vi "Test - Evaluation and Decoding.vi"() -> ()   [LabVIEW 2014, in "HMM.lvlib"]
uses:
  HMM.lvlib
panel:
  out "Beta Partial Probalility":dbl[][](array[numeric])
  out "Log10(Prob)":dbl
  out "Scale factor":dbl[](array[numeric])
  out "Probability - by forward scale":dbl
  out "Scaled Alpha":dbl[][](array[numeric])
  out "Possible Sequence":i32[](array[numeric])
  out "Probability - by backward":dbl
  out "backward Partial Probalility":dbl[][](array[numeric])
  out "forward Partial Probalility":dbl[][](array[numeric])
  in  "Observed Sequence":i32[](array[numeric])=[0, 2, 3]
  out "Probability - by forward":dbl
  in  "HMM Cluster":cluster{"A":dbl[][], "B":dbl[][], "Pi":dbl[]}={"A"=[[0.5, 0.375, 0.125], [0.25, 0.125, 0.625], [0.25, 0.375, 0.375]], "B"=[[0.6, 0.2, 0.15, 0.05], [0.25, 0.25, 0.25, 0.25], [0.05, 0.1, 0.35, 0.5]], "Pi"=[0.63, 0.17, 0.2]}
  # "Expected probability:\n0.0269014"
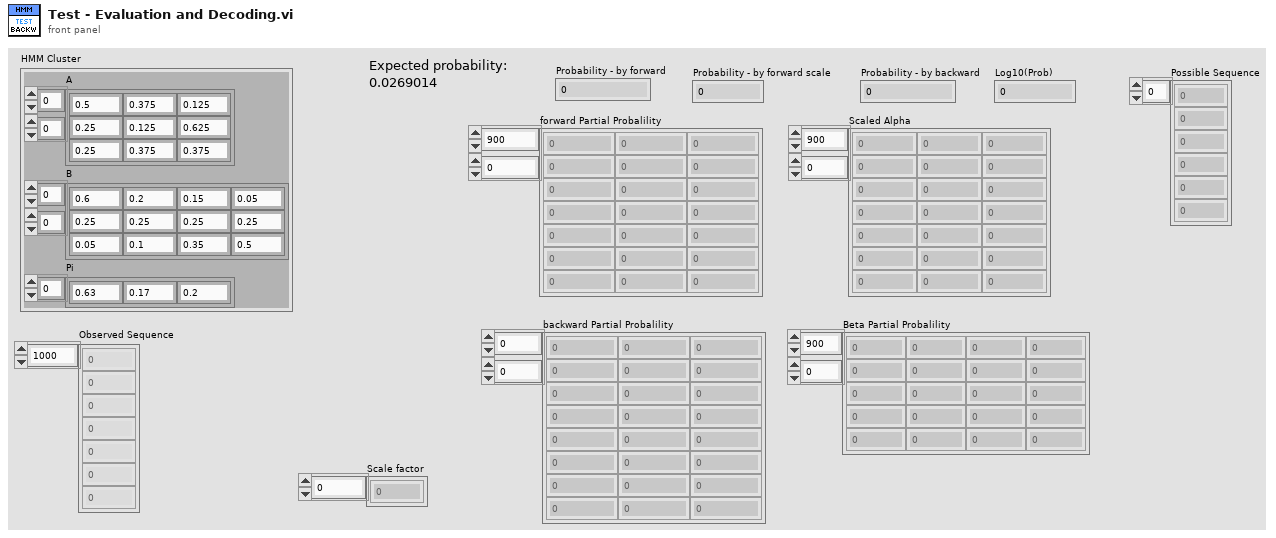
[diagram p1: front panel]
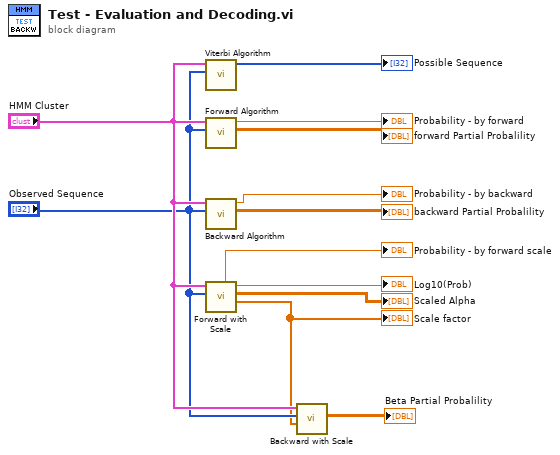
[diagram p0: block diagram]
diagram:
  n1 = call "Viterbi Algorithm.vi"("Observed Sequence"="Observed Sequence", "HMM Cluster"="HMM Cluster") -> ("Viterbi Path"=→"Possible Sequence":i32[])  [unwired: 8 in, 1 out]
  n2 = call "Forward Algorithm.vi"("O Observed Sequence"="Observed Sequence", "HMM Cluster"="HMM Cluster") -> ("Alpha Partial Probalility"=→"forward Partial Probalility":dbl[][], "Probability"=→"Probability - by forward":dbl)  [unwired: 8 in]
  n3 = call "Backward Algorithm.vi"("O Observed Sequence"="Observed Sequence", "HMM Cluster"="HMM Cluster") -> ("Beta Partial Probalility"=→"backward Partial Probalility":dbl[][], "Probability"=→"Probability - by backward":dbl)  [unwired: 8 in]
  n4 = call "Forward with Scale.vi"("O Observed Sequence"="Observed Sequence", "HMM Cluster"="HMM Cluster") -> ("Scale factor"=w4:dbl[], "Scaled Alpha"=→"Scaled Alpha":dbl[][], "Log10(Prob)"=→"Log10(Prob)":dbl, "Probability"=→"Probability - by forward scale":dbl)  [unwired: 6 in]
  "Scale factor" <- w4
  n5 = call "Backward with Scale.vi"("Scale factor"=w4, "O Observed Sequence"="Observed Sequence", "HMM Cluster"="HMM Cluster") -> ("Beta Partial Probalility"=→"Beta Partial Probalility":dbl[][])  [unwired: 8 in]
